vi "Setup 433x.vi"(8 "error in (no error)":errorcluster, 9 "SampleRate":dbl, 10 "task in":refnum<k21>) -> (0 "error out":errorcluster, 3 "433x":T1)   [LabVIEW 2011, in "PXIe-433x Custom Device.lvlib"]
uses:
  PXIe-433x Custom Device.lvlib
  433x data.ctl
  <vilib>/DAQmx/configure/timing.llb/DAQmx Timing (Sample Clock).vi
  Program Files (x86)/National Instruments/LabVIEW 2011/resource/objmgr/daqmx.rc
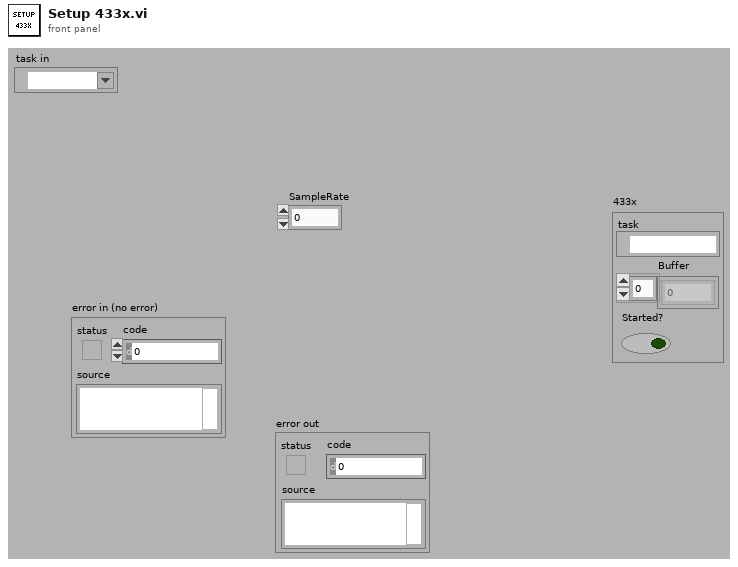
[diagram p1: front panel]
types:
  T1 = typedef "PXIe-433x Custom Device.lvlib/433x data.ctl" = cluster{"task":refnum<k21>, "Buffer":dbl[], "Started?":bool}
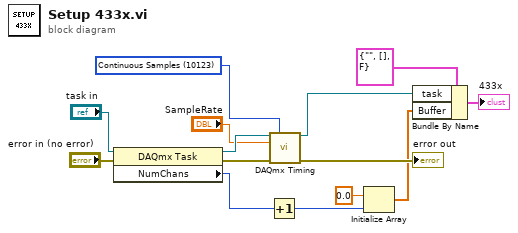
[diagram p0: block diagram]
diagram:
  w10 = 10123 items=["Finite Samples"=10178, "Continuous Samples"=10123] ("sample mode")
  n1 = property class="DAQmx Task"(reference="task in", error in="error in (no error)") -> (reference out=w12:refnum<k21>, error out=w13:errorcluster, "NumChans"=w7:u32)
  n2 = Increment(x=w7) -> (x+1=w3:u32)
  n3 = call-poly <vilib>:"DAQmx Timing.vi"("task/channels in"=w12, "sample mode"=w10, "rate"="SampleRate", "error in"=w13) -> ("task out"=w14:refnum<k21>, "error out"=→"error out":errorcluster)  [unwired: 10 in]
  n4 = Initialize Array(0.0 ("element"), w3) -> (w5:dbl[])
  n5 = Bundle By Name(cluster=T1 {"task"="", "Buffer"=[], "Started?"=FALSE} ("433x"), "task"=w14, "Buffer"=w5) -> (→"433x":T1)
